vi "test.vi"() -> ()   [LabVIEW 2014]
uses:
  Controls/XYPos.ctl
panel:
  out "点位示意图 2":T1(plugin-control)
  out "数组":cluster{"X":dbl, "Y":dbl}[](array[cluster])
  out "点位示意图":T1(plugin-control)
  out "添加的路径 2":path
  out "点位信息表":string[][](table)=[["PCB1-拍照点1(Mark1)", "-73.376", "-164.238", "0.000", "-103.848", "565.620", "384.924", "377.049", "0.000", "0.000", "0.000", "0", "8", "94", "1"], ["PCB1-拍照点2(Mark2)", "-260.376", "-49.239", "0.000", "-290.450", "681.264", "384.924", "377.049", "0.000", "0.000", "0.000", "-180", "8", "94", "1"], ["拍照点3", "-73.376", "-49.239", "0.000", "-103.451", "680.618", "384.924", "377.049", "0.000", "0.000", "0.000", "0", "8", "94", "1"], ["拍照点4", "-260.376", "-164.238", "0.000", "-290.847", "566.266", "384.924", "377.049", "0.000", "0.000", "0.000", "-180", "8", "94", "1"], ["拍照点5", "-260.376", "-104.239", "0.000", "-290.640", "626.265", "384.924", "377.049", "0.000", "0.000", "0.000", "-180", "8", "94", "1"], ["拍照点6", "-240.876", "-23.738", "0.000", "-270.862", "706.698", "384.924", "377.049", "0.000", "0.000", "0.000", "90", "8", "94", "1"], ["拍照点7", "-190.876", "-23.738", "0.000", "-220.862", "706.525", "384.924", "377.049", "0.000", "0.000", "0.000", "90", "8", "94", "0"], ["拍照点8", "-142.876", "-23.738", "0.000", "-172.862", "706.359", "384.924", "377.049", "0.000", "0.000", "0.000", "90", "8", "94", "0"], ["拍照点9", "-92.876", "-23.738", "0.000", "-122.863", "706.187", "384.924", "377.049", "0.000", "0.000", "0.000", "90", "8", "94", "0"], ["拍照点10", "-73.376", "-104.239", "0.000", "-103.641", "625.619", "384.924", "377.049", "0.000", "0.000", "0.000", "0", "8", "94", "0"], ["拍照点11", "-112.876", "-169.238", "0.000", "-143.365", "560.756", "384.924", "377.049", "0.000", "0.000", "0.000", "-90", "8", "94", "0"], ["拍照点12", "-220.876", "-169.238", "0.000", "-251.364", "561.130", "384.924", "377.049", "0.000", "0.000", "0.000", "0", "8", "94", "0"], ["PCB2-拍照点1(Mark3)", "-73.376", "-164.238", "0.000", "151.457", "565.201", "384.924", "377.049", "0.000", "0.000", "-3.000", "0", "8", "94", "1"], ["PCB2-拍照点2(Mark4)", "-260.376", "-49.239", "0.000", "-35.509", "680.255", "384.924", "377.049", "0.000", "0.000", "-3.000", "-180", "8", "94", "1"], ["拍照点3", "-73.376", "-49.239", "0.000", "151.491", "680.200", "384.924", "377.049", "0.000", "0.000", "-3.000", "0", "8", "94", "1"], ["拍照点4", "-260.376", "-164.238", "0.000", "-35.543", "565.256", "384.924", "377.049", "0.000", "0.000", "-3.000", "-180", "8", "94", "1"], ["拍照点5", "-260.376", "-104.239", "0.000", "-35.525", "625.255", "384.924", "377.049", "0.000", "0.000", "-3.000", "-180", "8", "94", "1"], ["拍照点6", "-240.876", "-23.738", "0.000", "-16.001", "705.751", "384.924", "377.049", "0.000", "0.000", "-3.000", "90", "8", "94", "1"], ["拍照点7", "-190.876", "-23.738", "0.000", "33.999", "705.736", "384.924", "377.049", "0.000", "0.000", "0.000", "90", "8", "94", "0"], ["拍照点8", "-142.876", "-23.738", "0.000", "81.999", "705.722", "384.924", "377.049", "0.000", "0.000", "0.000", "90", "8", "94", "0"], ["拍照点9", "-92.876", "-23.738", "0.000", "131.999", "705.707", "384.924", "377.049", "0.000", "0.000", "0.000", "90", "8", "94", "0"], ["拍照点10", "-73.376", "-104.239", "0.000", "151.475", "625.200", "384.924", "377.049", "0.000", "0.000", "0.000", "0", "8", "94", "0"], ["拍照点11", "-112.876", "-169.238", "0.000", "111.956", "560.213", "384.924", "377.049", "0.000", "0.000", "0.000", "-90", "8", "94", "0"], ["拍照点12", "-220.876", "-169.238", "0.000", "3.956", "560.245", "384.924", "377.049", "0.000", "0.000", "0.000", "0", "8", "94", "0"]]
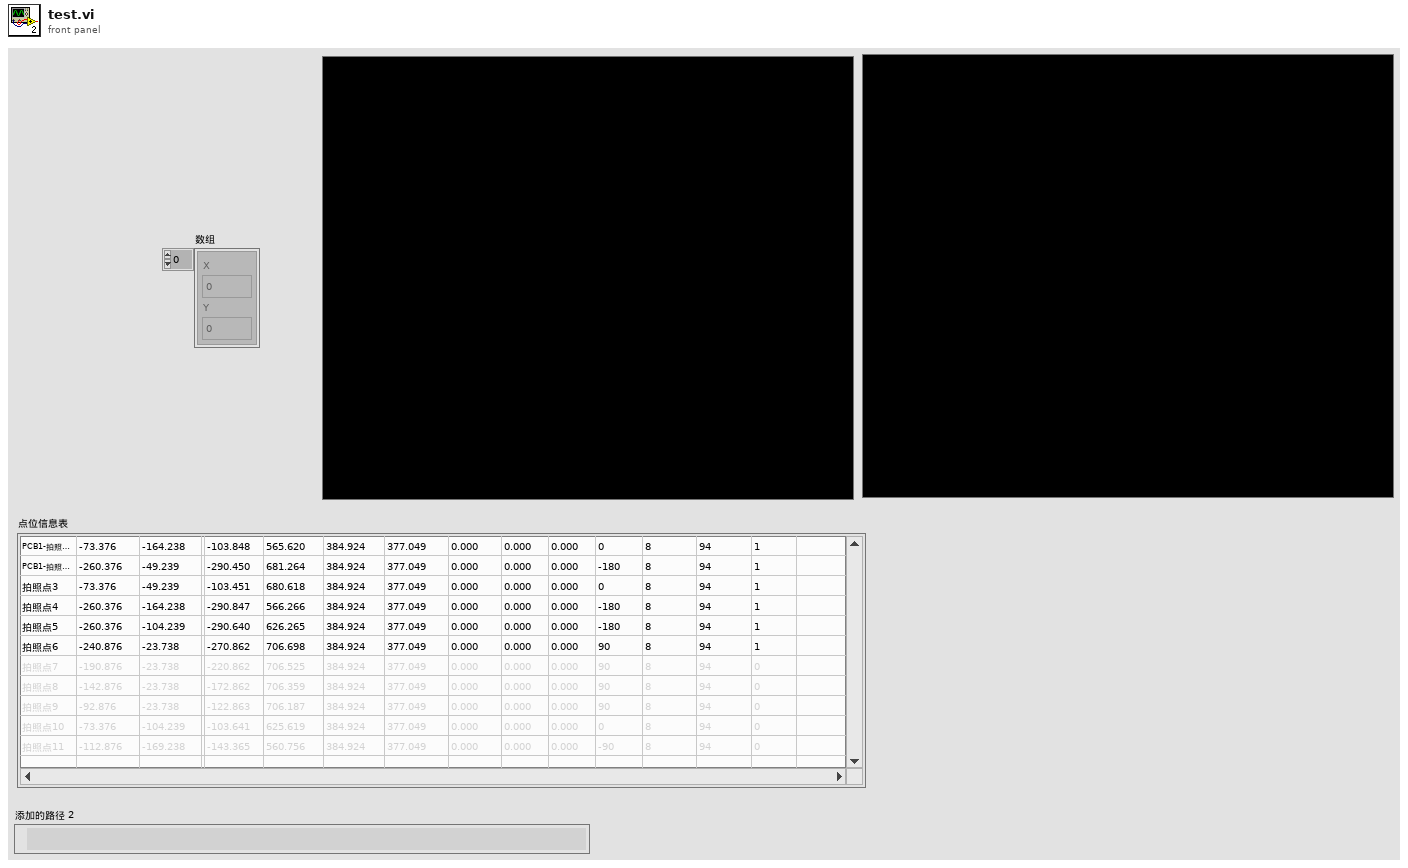
[diagram p1: front panel]
types:
  T1 = typedef "IMAQ Image.ctl" = refnum<image>
  T2 = typedef "Image Type" = u32
  T3 = typedef "控件-Excel读写选项.ctl" = enum16{"打开表格", "新增sheet", "读取sheet指定位置数据", "读取sheet整个数据", "写入sheet整个数据", "写表头", "数据存到本机", "表格是否开启状态", "关闭表格"}
  T4 = typedef "XYPos.ctl" = cluster{"X":dbl, "Y":dbl}
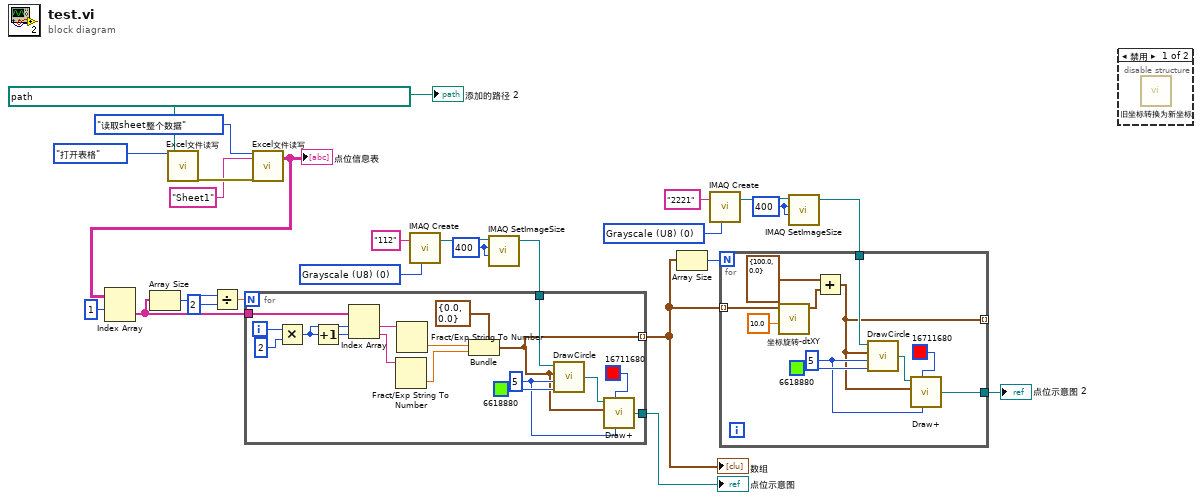
[diagram p0: block diagram]
diagram:
  w8 = 400 ("X Resolution")
  w6 = T2 0 items=["Grayscale (U8)", "Grayscale (I16)", "Grayscale (SGL)", "Complex (CSG)", "RGB (U32)", "HSL (U32)", "RGB (U64)", "Grayscale (U16)"] ("Image Type")
  w11 = 400 ("X Resolution")
  w13 = T2 0 items=["Grayscale (U8)", "Grayscale (I16)", "Grayscale (SGL)", "Complex (CSG)", "RGB (U32)", "HSL (U32)", "RGB (U64)", "Grayscale (U16)"] ("Image Type")
  w24 = path "E:/设备程序/王杰/光背板布线设备/光背板布线设备-20201021/1234.xlsx" ("file path (dialog if empty)")
  n1 = call "Excel文件读写.vi"("选项"=控件-Excel读写选项."打开表格", "Path"=w24) -> ("error out"=w23:errorcluster)  [unwired: 15 in, 2 out]
  n2 = call "Excel文件读写.vi"("选项"=控件-Excel读写选项."读取sheet整个数据", "sheet name"="Sheet1", "error in"=w23) -> ("data"=w15:string[][])  [unwired: 14 in, 2 out]
  "点位信息表" <- w15
  n3 = Index Array(array=w15, index (row)=1 ("索引 (行)")) -> (element=w17:string[])  [unwired: 1 in]
  n4 = Array Size(array=w17) -> (size(s)=w18:i32)
  n5 = Divide(x=w18, y=2) -> (x/y=w20:dbl)
  n6 = call "IMAQ Create"("Image Name"="112", "Image Type"=w13) -> ("New Image"=w12:T1)  [unwired: 3 in, 1 out]
  n7 = call "IMAQ SetImageSize"("Y Resolution"=w11, "X Resolution"=w11, "Image"=w12) -> ("Image Out"=w10:T1)  [unwired: 2 in, 1 out]
  n8 = for {
    N: w20 -> [_]
    tunnel: w17 -> [w42]
    tunnel: w10 -> [w32]
    tunnel: [w28] -> w9
    tunnel: [w26] -> w1 mode=indexing
    i -> [w41]
    w30 = 5 ("Circle_D")
    n9 = Multiply(x=w41, y=2) -> (x*y=w39:i32)
    n10 = Increment(x=w39) -> (x+1=w38:i32)
    n11 = Index Array(array=w42, index #1=w39, index #2=w38) -> (element #1=w37:string, element #2=w36:string)
    n12 = Fract/Exp String To Number(string=w36) -> (number=w34:dbl)  [unwired: 3 in, 1 out]
    n13 = Fract/Exp String To Number(string=w37) -> (number=w35:dbl)  [unwired: 3 in, 1 out]
    n14 = Bundle(cluster=cluster{"X":dbl, "Y":dbl} {"X"=0.0, "Y"=0.0}, "X"=w35, "Y"=w34) -> (w26:cluster{"X":dbl, "Y":dbl})
    n15 = call "DrawCircle.vi"("Color"=u32 6618880, "Circle_D"=w30, "CircleCenterPosition"=w26, "Img in"=w32) -> ("Img out"=w29:T1)
    n16 = call "Draw+.vi"("Width"=w30, "Color"=u32 16711680, "input cluster"=w26, "Image In"=w29) -> ("Image Out"=w28:T1)  [unwired: 2 in]
  }
  "点位示意图" <- w9
  "数组" <- w1
  n17 = Array Size(array=w1) -> (size(s)=w2:i32)
  n18 = call "IMAQ Create"("Image Name"="2221", "Image Type"=w6) -> ("New Image"=w7:T1)  [unwired: 3 in, 1 out]
  n19 = call "IMAQ SetImageSize"("Y Resolution"=w8, "X Resolution"=w8, "Image"=w7) -> ("Image Out"=w4:T1)  [unwired: 2 in, 1 out]
  n20 = for {
    N: w2 -> [_]
    tunnel: [w44] -> _ mode=indexing
    tunnel: [w48] -> w3
    tunnel: w4 -> [w47]
    tunnel: w1 -> [w46] mode=indexing
    w49 = 5 ("Circle_D")
    n21 = call "坐标旋转-dtXY.vi"("旋转角度(单位角度)"=10.0, "dtx,dty In"=w46) -> ("dtx,dty Out"=w45:T4)  [unwired: 9 in]
    n22 = Add(x=T4 {"X"=100.0, "Y"=0.0}, y=w45) -> (x+y=w44:T4)
    n23 = call "DrawCircle.vi"("Color"=u32 6618880, "Circle_D"=w49, "CircleCenterPosition"=w44, "Img in"=w47) -> ("Img out"=w51:T1)
    n24 = call "Draw+.vi"("Width"=w49, "Color"=u32 16711680, "input cluster"=w44, "Image In"=w51) -> ("Image Out"=w48:T1)  [unwired: 2 in]
  }
  "点位示意图 2" <- w3
  n25 = disable-structure shown="禁用" {
    frame Disabled {
      n26 = call "旧坐标转换为新坐标.vi"() -> ()  [unwired: 4 in, 1 out]
    }
    frame Enabled {
    }
  }
  "添加的路径 2" <- w24
